vi "VI_Center_Control.vi"(7 "force maximize Frontpanel?":bool, 8 "Error In":errorcluster, 10 "Target Ctl Refnum (In)":refnum<vi>, 11 "VI Refnum (In)":refnum<vi>) -> (0 "Error Out":errorcluster)   [LabVIEW 2014]
uses:
  <vilib>/Utility/miscctls.llb/LVPositionTypeDef.ctl
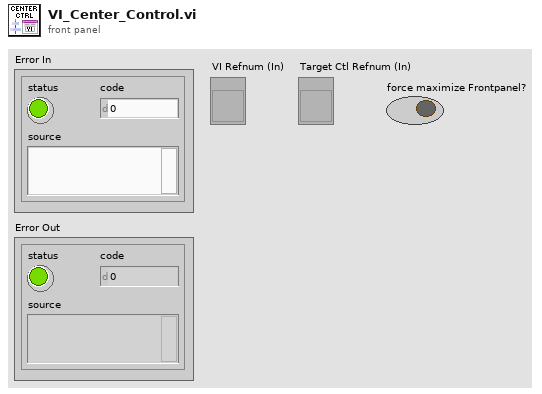
[diagram p1: front panel]
types:
  T1 = typedef "LVPositionTypeDef.ctl" = cluster{"Left":i32, "Top":i32}
  T2 = enum32{"Invalid", "Standard", "Closed", "Hidden", "Minimized", "Maximized"}
  T3 = typedef "LVRectTypeDef.ctl" = cluster{"Left":i16, "Top":i16, "Right":i16, "Bottom":i16}
  T4 = typedef "LVBoundsTypeDef.ctl" = cluster{"Width":u32, "Height":u32}
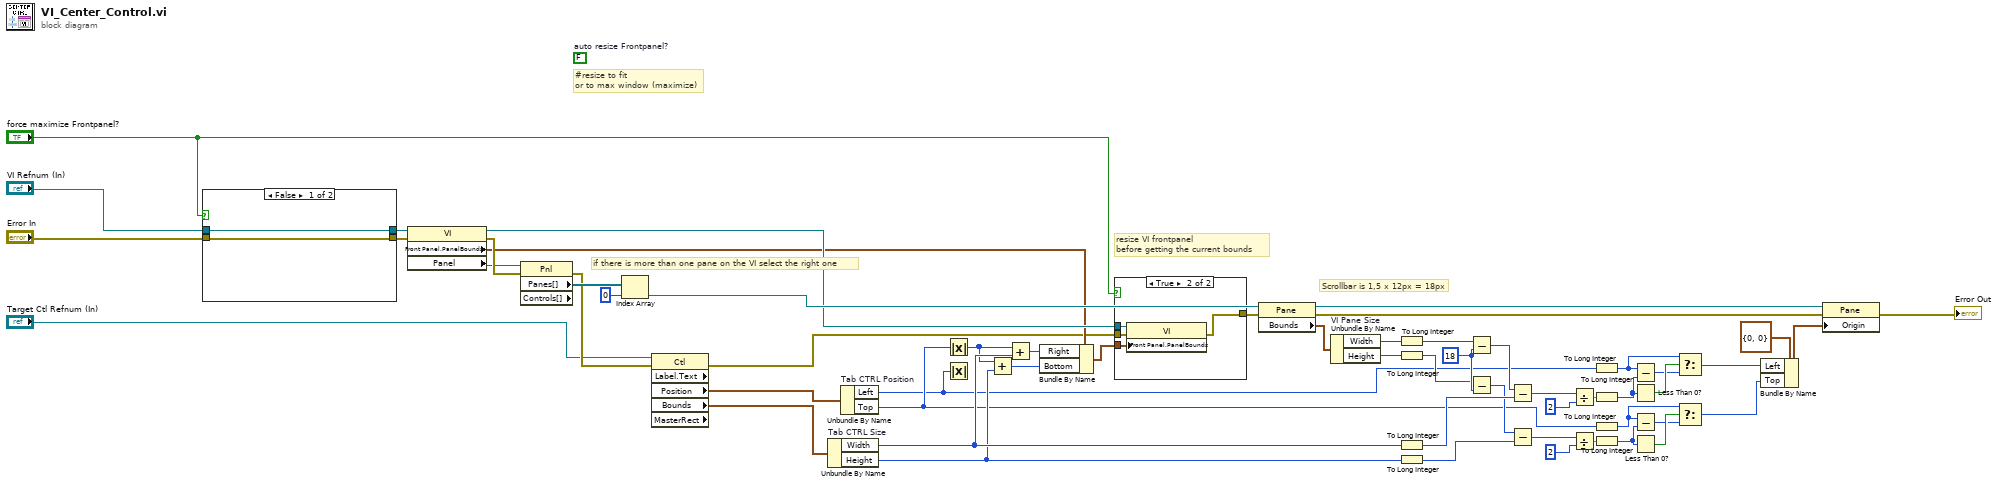
[diagram p0: block diagram]
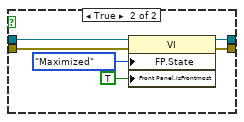
[diagram p3: hidden frame]
diagram:
  w28 = 18
  (unwired) FALSE  # auto resize Frontpanel?
  # "if there is more than one pane on the VI select the right one"
  # "resize VI frontpanel\nbefore getting the current bounds"
  # "#resize to fit\nor to max window (maximize)"
  # "Scrollbar is 1,5 x 12px = 18px"
  n1 = case shown="False" "force maximize Frontpanel?" {
    tunnel: "Error In" -> [w58 w65]
    tunnel: "VI Refnum (In)" -> [w59 w64]
    tunnel: [w58 w61] -> w13
    tunnel: [w59 w60] -> w3
    frame False {
    }
    frame True {
      n2 = property class="VI"(reference=w64, error in=w65, "FP.State"=T2."Maximized" ("Front Panel Window:State"), "Front Panel.IsFrontmost"=TRUE ("Front Panel Window:Is Frontmost")) -> (reference out=w60:refnum<vi>, error out=w61:errorcluster)
    }
  }
  n3 = property class="VI"(reference=w3, error in=w13) -> (reference out=w12:refnum<vi>, error out=w22:errorcluster, "Front Panel.PanelBounds"=w11:T3, "Panel"=w2:refnum<vi>)
  n4 = property class="Pnl" props=["Panes[]", "Controls[]"](reference=w2, error in=w22) -> (error out=w50:errorcluster, "Panes[]"=w57:refnum<vi>[])  [unwired: 2 out]
  n5 = Index Array(array=w57, index=0) -> (element=w24:refnum<vi>)
  n6 = property class="Ctl" props=["Label", "Text", "Position", "Bounds", "MasterRect"](reference="Target Ctl Refnum (In)", error in=w50) -> (error out=w9:errorcluster, "Position"=w56:T1, "Bounds"=w55:T4)  [unwired: 3 out]
  n7 = Unbundle By Name "Tab CTRL Size"(w55) -> ("Width"=w19:u32, "Height"=w18:u32)
  n8 = Unbundle By Name "Tab CTRL Position"(w56) -> ("Left"=w15:i32, "Top"=w16:i32)
  n9 = Absolute Value(x=w16) -> (abs(x)=w17:i32)
  n10 = Absolute Value(x=w15) -> ()  [unwired: 1 out]
  n11 = Add(x=w17, y=w18) -> (x+y=w20:u32)
  n12 = Add(x=w17, y=w19) -> (x+y=w21:u32)
  n13 = Bundle By Name(cluster=w11, "Right"=w21, "Bottom"=w20) -> (w14:T3)
  n14 = case shown="True" "force maximize Frontpanel?" {
    tunnel: w14 -> [_ w70]
    tunnel: w12 -> [_ w69]
    tunnel: [w66 w68] -> w10
    tunnel: w9 -> [w66 w67]
    frame False {
    }
    frame True {
      n15 = property class="VI"(reference=w69, error in=w67, "Front Panel.PanelBounds"=w70) -> (error out=w68:errorcluster)  [unwired: 1 out]
    }
  }
  n16 = property class="Pane"(reference=w24, error in=w10) -> (reference out=w23:refnum<vi>, error out=w51:errorcluster, "Bounds"=w52:T4)
  n17 = Unbundle By Name "VI Pane Size"(w52) -> ("Width"=w40:u32, "Height"=w43:u32)
  n18 = To Long Integer(number=w40) -> (32bit integer=w31:i32)
  n19 = To Long Integer(number=w43) -> (32bit integer=w27:i32)
  n20 = To Long Integer(number=w19) -> (32bit integer=w41:i32)
  n21 = To Long Integer(number=w18) -> (32bit integer=w42:i32)
  n22 = Subtract(x=w31, y=w28) -> (x-y=w30:i32)
  n23 = Subtract(x=w27, y=w28) -> (x-y=w29:i32)
  n24 = Subtract(x=w30, y=w41) -> (x-y=w47:i32)
  n25 = Subtract(x=w29, y=w42) -> (x-y=w46:i32)
  n26 = Divide(x=w47, y=2) -> (x/y=w44:dbl)
  n27 = Divide(x=w46, y=2) -> (x/y=w45:dbl)
  n28 = To Long Integer(number=w15) -> (32bit integer=w34:i32)
  n29 = To Long Integer(number=w44) -> (32bit integer=w36:i32)
  n30 = To Long Integer(number=w16) -> (32bit integer=w26:i32)
  n31 = To Long Integer(number=w45) -> (32bit integer=w25:i32)
  n32 = Subtract(x=w34, y=w36) -> (x-y=w33:i32)
  n33 = Less Than 0?(x=w36) -> (x < 0?=w35:bool)
  n34 = Subtract(x=w26, y=w25) -> (x-y=w37:i32)
  n35 = Less Than 0?(x=w25) -> (x < 0?=w39:bool)
  n36 = Select(t=w34, s=w35, f=w33) -> (s? t:f=w32:i32)
  n37 = Select(t=w26, s=w39, f=w37) -> (s? t:f=w38:i32)
  n38 = Bundle By Name(cluster=T1 {"Left"=0, "Top"=0} ("Position"), "Left"=w32, "Top"=w38) -> (w53:T1)
  n39 = property class="Pane"(reference=w23, error in=w51, "Origin"=w53) -> (error out=→"Error Out":errorcluster)  [unwired: 1 out]
